vi "setUp.vi"(8 "error in (no error)":errorcluster, 11 "reference in":refnum<class "Instrument Addon Error System Tests.lvclass">) -> (0 "error out":errorcluster, 3 "reference out":refnum<class "Instrument Addon Error System Tests.lvclass">)   [LabVIEW 2019, in "Instrument Addon Error System Tests.lvclass"]
doc: "setUp runs prior to the test method during test execution. Use this method to initialize any object data required by your tests."
uses:
  Instrument Addon Error System Tests.lvclass
  C:/Program Files (x86)/National Instruments/LabVIEW 2019/vi.lib/NI/VeriStand Custom Device Testing Tools/VeriStandTestCase/VeriStandTestCase.lvclass
  C:/Program Files (x86)/National Instruments/LabVIEW 2019/vi.lib/addons/_JKI Toolkits/VI Tester/TestCase.llb/TestCase.lvclass
  <vilib>/NI VeriStand/Execution/Workspace/NI VeriStand - Set Multiple Channel Values.vi
  <vilib>/addons/_JKI Toolkits/VI Tester/TestCase.llb/TestCase.lvclass
  <vilib>/NI VeriStand/Execution/Workspace/NI_VS Workspace ExecutionAPI.lvlib
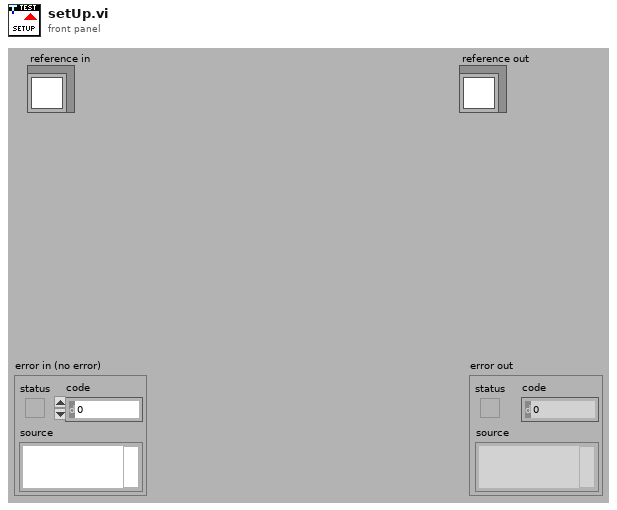
[diagram p1: front panel]
types:
  T1 = typedef "NI_VS Workspace ExecutionAPI.lvlib/WorkspaceAPI.ctl" = refnum<k24>
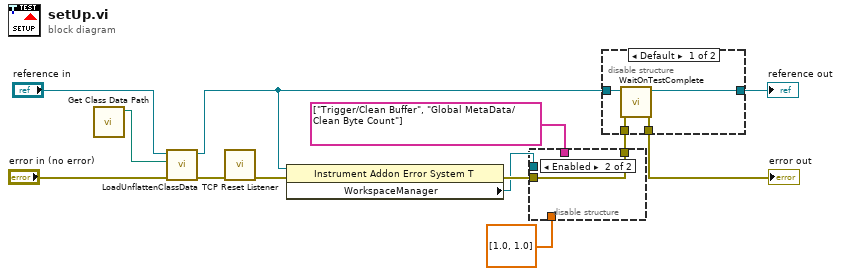
[diagram p0: block diagram]
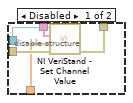
[diagram p2: hidden frame]
diagram:
  n1 = call "Get Class Data Path.vi"() -> ("Class Data File Path"=w9:path)  [unwired: 11 in]
  n2 = call-dynamic "LoadUnflattenClassData.vi"("error in"="error in (no error)", "Class Data File Path"=w9, "VeriStandTestCase in"="reference in") -> ("error out"=w8:errorcluster, "VeriStandTestCase out"=w7:refnum<class "Instrument Addon Error System Tests.lvclass">)  [unwired: 7 in]
  n3 = call "TCP Reset Listener.vi"("error in (no error)"=w8) -> ("error out"=w6:errorcluster)  [unwired: 10 in]
  n4 = property class="Instrument Addon Error System T"(reference=w7, error in=w6) -> (error out=w5:errorcluster, "WorkspaceManager"=w3:T1)  [unwired: 1 out]
  n5 = disable-structure shown="Enabled" {
    disable-tunnel: w5 -> [w18 w19]
    disable-tunnel: string[] ["Trigger/Clean Buffer", "Global MetaData/Clean Byte Count"] ("Channel Alias") -> [w17 _]
    disable-tunnel: w3 -> [w16 _]
    disable-tunnel: [w15 w19] -> w2
    disable-tunnel: dbl[] [1.0, 1.0] ("Values") -> [w14 _]
    frame Disabled {
      n6 = call-poly <vilib>:"NI VeriStand - Set Channel Value.vi"("error in (no error)"=w18, "Values"=w14, "Channels"=w17, "WorkspaceManager in"=w16) -> ("error out"=w15:errorcluster)  [unwired: 6 in, 1 out]
    }
    frame Enabled {
    }
  }
  n7 = disable-structure shown="Default" {
    disable-tunnel: w2 -> [w23 w24]
    disable-tunnel: [w22 w24] -> w13
    disable-tunnel: [w21 w25] -> w12
    disable-tunnel: w7 -> [w20 w25]
    frame condition #0 (active) {
      n8 = call <vilib>:"WaitOnTestComplete.vi"("error in (no error)"=w23, "TestCase in"=w20) -> ("error out"=w22:errorcluster, "TestCase out"=w21:refnum<class "Instrument Addon Error System Tests.lvclass">)  [unwired: 8 in]
    }
    frame condition #1 {
    }
  }
  "error out" <- w13
  "reference out" <- w12
